vi "Requests.vi"(8 "error in (no error)":errorcluster, 9 "write enable":bool=TRUE, 11 "ICPCON ET in":refnum<class "ICPCON ET-7024ao.lvclass">) -> (0 "error out":errorcluster, 3 "ICPCON ET out":refnum<class "ICPCON ET-7024ao.lvclass">)   [LabVIEW 2019, in "ICPCON ET-7024ao.lvclass"]
uses:
  ICPCON ET-7024ao.lvclass
  D:/my_projects/projects/Algorithms/Labview/19/Modbus/MB_TCP2/MB_TCP.lvclass
  MB_TCP.lvclass/MB_TCP.ctl
  NI_modbus_upd/Ctl/Unit_ID.ctl
  NI_modbus_upd/TCP/TCP.lvclass/TCP.ctl
  NI_modbus_upd/Master Function Definition/Responses/Read Discrete Inputs Response.vi
  NI_modbus_upd/Master network read write.vi
  NI_modbus_upd/Master Function Definition/Requests/Read Discrete Inputs Request.vi
  NI_modbus_upd/Master Function Definition/Responses/Read Coils Response.vi
  NI_modbus_upd/Master Function Definition/Requests/Read Coils Request.vi
  NI_modbus_upd/Master Function Definition/Responses/Read Holding Registers Response.vi
  NI_modbus_upd/Master Function Definition/Requests/Read Holding Registers Request.vi
  NI_modbus_upd/Function data mismatch error1.vi
  NI_modbus_upd/Master Function Definition/Responses/Write Multiple Registers Response.vi
  NI_modbus_upd/Master Function Definition/Requests/Write Multiple Registers Request.vi
  NI_modbus_upd/Utility/Bytes to Bits1.vi
  NI_modbus_upd/Function code mismatch error1.vi
  NI_modbus_upd/Error Generator1.vi
  NI_modbus_upd/Read ADU Packet Master.vi
  NI_modbus_upd/Write ADU Packet Master.vi
  NI_modbus_upd/Modbus Data Unit (PDU)/Construct PDU1.vi
  NI_modbus_upd/Utility/Bytes to U16s1.vi
  NI_modbus_upd/Utility/U16s to Bytes1.vi
  NI_modbus_upd/Modbus Data Unit (PDU)/Unflatten to PDU1.vi
  NI_modbus_upd/TCP/Protocol Read.vi
  NI_modbus_upd/TCP/Protocol Write.vi
  <vilib>/Utility/error.llb/Clear Errors.vi
  NI_modbus_upd/Modbus Data Unit (PDU)/Deconstruct PDU1.vi
  NI_modbus_upd/TCP/TCP.lvclass
  ICPCON Registers/ICPCON Registers.lvlib
  MB_TCP.lvclass
  NI_modbus_upd/NI_modbus_upd.lvlib
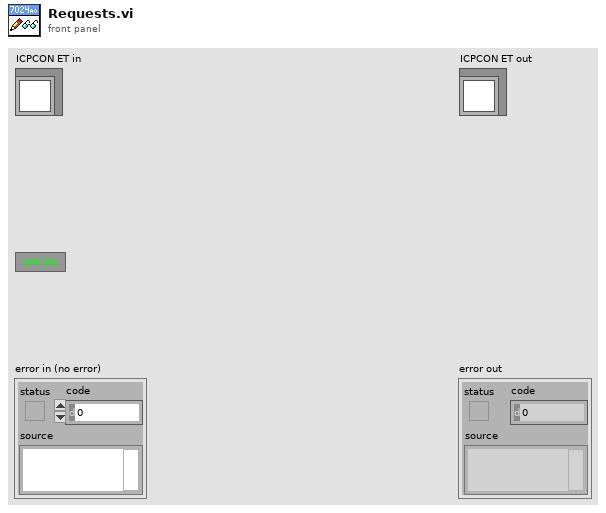
[diagram p1: front panel]
types:
  T1 = typedef "NI_modbus_upd.lvlib/Unit_ID.ctl" = cluster{"Protocol ID":u16, "Unit ID":u8}
  T2 = typedef "ICPCON Registers.lvlib/ICPCON Data.ctl" = cluster{"UTF":refnum<data-value>, "DI":refnum<data-value>, "DW":refnum<data-value>, "DO":refnum<data-value>, "IR":refnum<data-value>, "WR":refnum<data-value>, "OR":refnum<data-value>, "modified":refnum<data-value>}
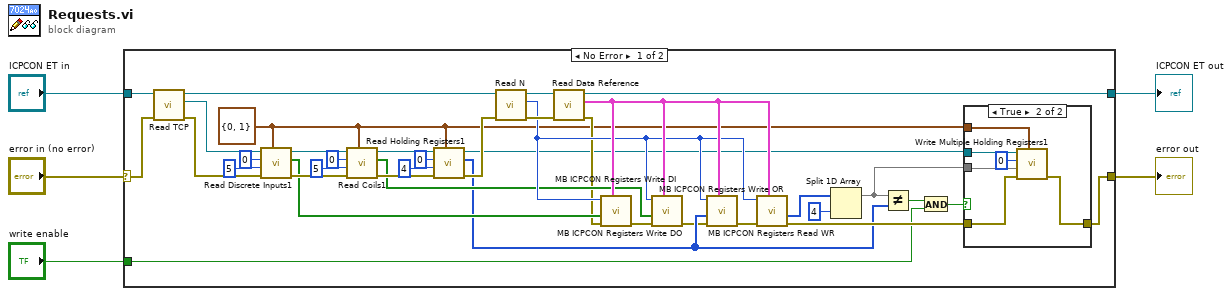
[diagram p0: block diagram]
diagram:
  n1 = case shown="No Error" "error in (no error)" {
    selector: "error in (no error)" -> [w26 w52]
    tunnel: [w17 w52] -> w3
    tunnel: [w24 w51] -> w4
    tunnel: "ICPCON ET in" -> [w27 w51]
    tunnel: "write enable" -> [w12 _]
    frame No Error {
      w8 = T1 {"Protocol ID"=0, "Unit ID"=1} ("Unit_ID")
      n2 = call "Read TCP.vi"("error in (no error)"=w26, "MB_TCP in"=w27) -> ("error out"=w31:errorcluster, "TCP"=w33:refnum<class "TCP.lvclass">, "MB_TCP out"=w32:refnum<class "ICPCON ET-7024ao.lvclass">)  [unwired: 7 in]
      n3 = call "Read Discrete Inputs1.vi"("Unit_ID"=w8, "error in (no error)"=w31, "number of discrete inputs"=u16 5, "starting address"=u16 0, "Modbus master in"=w33) -> ("error out"=w34:errorcluster, "discrete input values"=w28:bool[], "Modbus master out"=w30:refnum<class "TCP.lvclass">)  [unwired: 4 in]
      n4 = call "Read Coils1.vi"("Unit_ID"=w8, "error in (no error)"=w34, "number of coils"=u16 5 ("number of discrete inputs"), "starting address"=u16 0, "Modbus master in"=w30) -> ("error out"=w37:errorcluster, "coil values"=w13:bool[], "Modbus master out"=w29:refnum<class "TCP.lvclass">)  [unwired: 4 in]
      n5 = call "Read Holding Registers1.vi"("Unit_ID"=w8, "error in (no error)"=w37, "number of holding registers"=u16 4 ("number of discrete inputs"), "starting address"=u16 0, "Modbus master in"=w29) -> ("error out"=w25:errorcluster, "register values"=w10:u16[], "Modbus master out"=w7:refnum<class "TCP.lvclass">)  [unwired: 4 in]
      n6 = call "Read N.vi"("error in (no error)"=w25, "MB_TCP in"=w32) -> ("error out"=w42:errorcluster, "N"=w14:i32, "MB_TCP out"=w43:refnum<class "ICPCON ET-7024ao.lvclass">)  [unwired: 7 in]
      n7 = call "Read Data Reference.vi"("error in (no error)"=w42, "MB_TCP in"=w43) -> ("error out"=w9:errorcluster, "Data"=w15:T2, "MB_TCP out"=w24:refnum<class "ICPCON ET-7024ao.lvclass">)  [unwired: 7 in]
      n8 = call "MB ICPCON Registers Write DI.vi"("Data Reference"=w15, "error in (no error)"=w9, "Bits In"=w28, "N"=w14) -> ("error out"=w11:errorcluster)  [unwired: 7 in]
      n9 = call "MB ICPCON Registers Write DO.vi"("Data Reference"=w15, "error in (no error)"=w11, "Bits In"=w13, "N"=w14) -> ("error out"=w6:errorcluster)  [unwired: 7 in]
      n10 = call "MB ICPCON Registers Write OR.vi"("Data Reference"=w15, "error in (no error)"=w6, "Words In"=w10, "N"=w14) -> ("error out"=w16:errorcluster)  [unwired: 7 in]
      n11 = call "MB ICPCON Registers Read WR.vi"("Data Reference"=w15, "error in (no error)"=w16, "N"=w14) -> ("error out"=w18:errorcluster, "Words out"=w22:u16[])  [unwired: 7 in]
      n12 = Split 1D Array(array=w22, index=4 ("length")) -> (first subarray=w19:u16[])  [unwired: 1 out]
      n13 = Not Equal?(x=w19, y=w10) -> (x != y?=w21:bool)
      n14 = And(x=w21, y=w12) -> (x .and. y?=w20:bool)
      n15 = case shown="True" w20 {
        tunnel: w18 -> [w44 w49]
        tunnel: [w44 w47] -> w17
        tunnel: w7 -> [_ w50]
        tunnel: w8 -> [_ w45]
        tunnel: w19 -> [_ w46]
        frame False {
        }
        frame True {
          n16 = call "Write Multiple Holding Registers1.vi"("Unit_ID"=w45, "error in (no error)"=w49, "holding register values"=w46, "starting address"=u16 0, "Modbus master in"=w50) -> ("error out"=w47:errorcluster)  [unwired: 5 in, 1 out]
        }
      }
    }
    frame Error {
    }
  }
  "error out" <- w3
  "ICPCON ET out" <- w4
